vi "SRV_Motors Config Buttons MAP.vi"() -> (0 "error out":errorcluster)   [LabVIEW 2014]
doc: "A Producer-Consumer two-loop state machine template. This template uses the LPD Command Queues to drive its execution.\n\nThere are several advantages such as:\n- convenient error state control\n- the ability to pass data between states/loops/VIs via a variant\n- command history which is extremely valuable in troubleshooting when an error occurs\n\n\nAuthor: Mike Schultz\n\nLogicPD, Inc\nwww.logicpd.com"
uses:
  Support/SRV_Command-Data Queue Data Type.ctl
panel:
  in  "CLOSE":bool
  # "436x250"
  # "672x216"
  # "666x214"
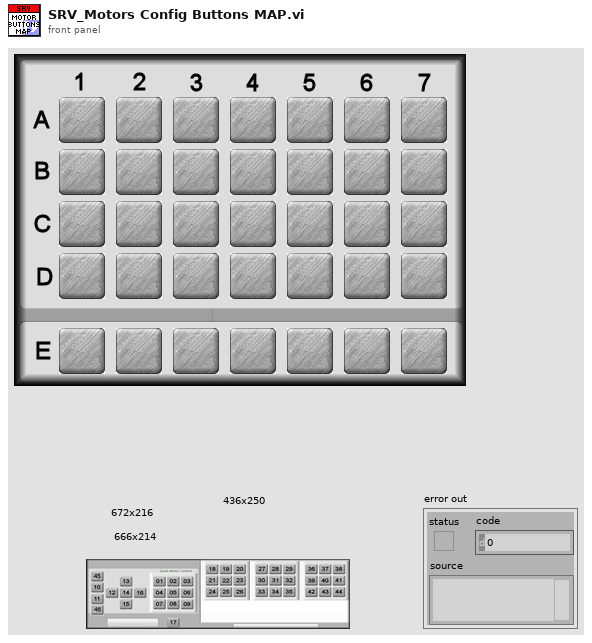
[diagram p1: front panel]
types:
  T1 = typedef "SRV_Command-Data Queue Data Type.ctl" = cluster{"Command":string, "Data":variant}
  T2 = cluster{"user event":refnum<user-event>, "VI ref":refnum<vi>}
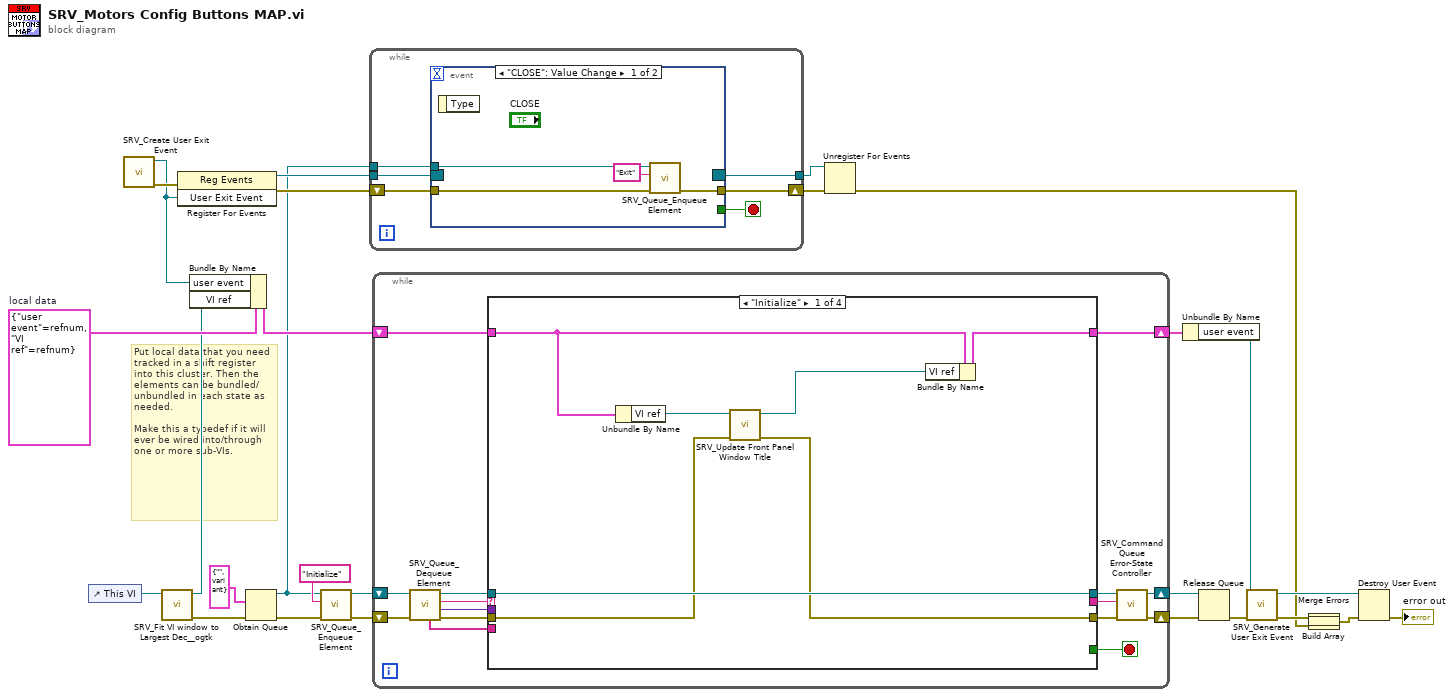
[diagram p0: block diagram]
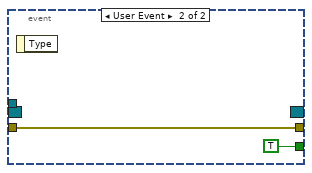
[diagram p2: hidden frame]
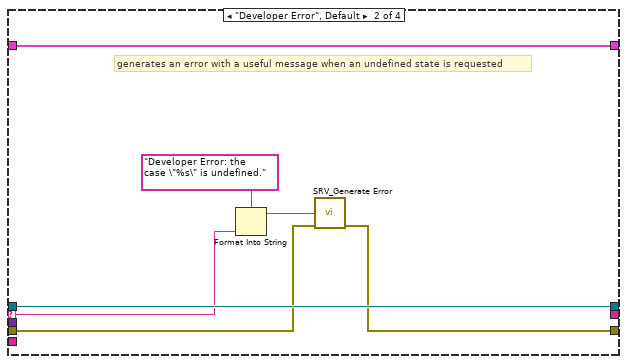
[diagram p3: hidden frame]
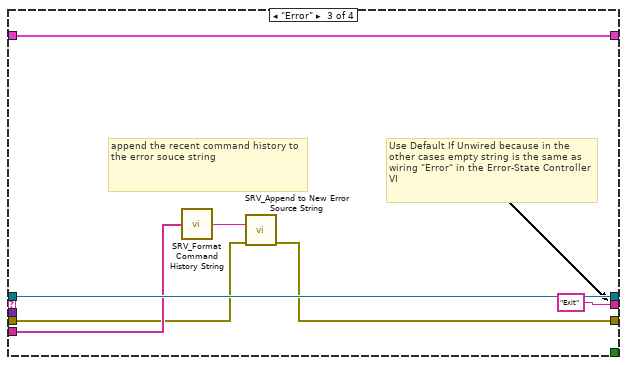
[diagram p4: hidden frame]
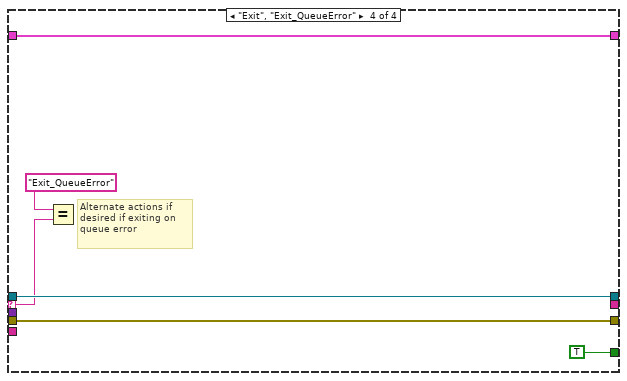
[diagram p5: hidden frame]
diagram:
  w21 = T2 {"user event"=refnum, "VI ref"=refnum}  # local data
  # "Put local data that you need tracked in a shift register into this cluster. Then the elements can be bundled/unbundled in each state as needed.\n\nMake this a typedef if it will ever be wired into/through one or more sub-VIs."
  n1 = control-ref of="This VI"() -> (w2:refnum<vi>)
  n2 = call "SRV_Create User Exit Event.vi"() -> ("error out"=w12:errorcluster, "User Exit Event"=w11:refnum<user-event>)  [unwired: 10 in]
  n3 = call "SRV_Fit VI window to Largest Dec__ogtk.vi"("VI Ref (calling VI)"=w2) -> ("error out"=w5:errorcluster, "dup VI Ref"=w1:refnum<vi>)  [unwired: 5 in]
  n4 = register-events(error in=w12, w11) -> (reference out=w28:refnum<event-registration>, error out=w27:errorcluster)  [unwired: 1 in]
  n5 = Bundle By Name(cluster=w21, "user event"=w11, "VI ref"=w1) -> (w20:T2)
  n6 = Obtain Queue(element data type=T1 {"Command"="", "Data"=variant} ("Queue Data Type"), error in (no error)=w5) -> (queue out=w7:refnum<queue>, error out=w8:errorcluster)  [unwired: 3 in, 1 out]
  n7 = call "SRV_Queue_Enqueue Element.vi"("error in (no error)"=w8, "Command"="Initialize", "Command-Data Queue"=w7) -> ("error out"=w3:errorcluster, "Command-Data Queue out"=w6:refnum<queue>)  [unwired: 6 in, 1 out]
  n8 = while {
    shift-right: [w33] -> w25
    shift-left: w27 -> [w34]
    tunnel: w7 -> [w32]
    tunnel: w28 -> [w31]
    tunnel: [w30] -> w26
    stop <- w29 stop-if-true
    n9 = event shown="[0] \"CLOSE\": Value Change" {
      selector: w31 -> [_ _]
      dyn-events: [_ _] -> w30
      timeout: _ -> [_ _]
      tunnel: w34 -> [w36 w40]
      tunnel: [w37 w40] -> w33
      tunnel: w32 -> [w35 _]
      tunnel: [_ TRUE] -> w29
      event "CLOSE": Value Change {
        n10 = event-data() -> ()  [unwired: 1 in, 1 out]
        n11 = call "SRV_Queue_Enqueue Element.vi"("error in (no error)"=w36, "Command"="Exit", "Command-Data Queue"=w35) -> ("error out"=w37:errorcluster)  [unwired: 6 in, 2 out]
      }
      event User Event {
        n12 = event-data() -> ()  [unwired: 1 in, 1 out]
      }
    }
  }
  n13 = while {
    shift-right: [w49] -> w24
    shift-left: w3 -> [w55]
    shift-right: [w47] -> w23
    shift-left: w6 -> [w53]
    shift-right: [w41] -> w19
    shift-left: w20 -> [w42]
    stop <- w43 stop-if-true
    n14 = call "SRV_Queue_Dequeue Element.vi"("error in (no error)"=w55, "Command-Data Queue"=w53) -> ("error out"=w54:errorcluster, "Data"=w46:variant, "Command"=w51:string, "Command-Data Queue out"=w52:refnum<queue>, "Command History"=w45:string[])  [unwired: 4 in, 1 out]
    n15 = case shown="\"Initialize\"" w51 {
      selector: w51 -> [_ w67 _ w79]
      tunnel: w54 -> [w61 w65 w71 w81]
      tunnel: [w60 w64 w72 w81] -> w50
      tunnel: w52 -> [w62 w69 w76 w82]
      tunnel: [w62 w69 w76 w82] -> w48
      tunnel: w46 -> [_ _ _ _]
      tunnel: w45 -> [_ _ w75 _]
      tunnel: [_ _ "Exit" ("Error Command") _] -> w44
      tunnel: [_ _ _ TRUE] -> w43
      tunnel: w42 -> [w58 w66 w73 w77]
      tunnel: [w57 w66 w73 w77] -> w41
      frame "Initialize" {
        n16 = Unbundle By Name(w58) -> ("VI ref"=w59:refnum<vi>)
        n17 = call "SRV_Update Front Panel Window Title.vi"("error in (no error)"=w61, "VI ref"=w59) -> ("error out"=w60:errorcluster, "VI ref out"=w56:refnum<vi>)  [unwired: 8 in]
        n18 = Bundle By Name(cluster=w58, "VI ref"=w56) -> (w57:T2)
      }
      frame "Developer Error", Default {
        # "generates an error with a useful message when an undefined state is requested"
        n19 = Format Into String(format string="Developer Error: the case \"%s\" is undefined.", w67) -> (resulting string=w63:string)  [unwired: 2 in, 1 out]
        n20 = call "SRV_Generate Error.vi"("Message"=w63, "error in (no error)"=w65) -> ("error out"=w64:errorcluster)  [unwired: 13 in]
      }
      frame "Error" {
        # "Use Default If Unwired because in the other cases empty string is the same as wiring \"Error\" in the Error-State Controller VI"
        # "append the recent command history to the error souce string"
        n21 = call "SRV_Format Command History String.vi"("Command History"=w75) -> ("Command History String"=w70:string)  [unwired: 14 in]
        n22 = call "SRV_Append to New Error Source String.vi"("Message String to append"=w70, "Error In (no error)"=w71) -> ("error out"=w72:errorcluster)  [unwired: 13 in]
      }
      frame "Exit", "Exit_QueueError" {
        # "Alternate actions if desired if exiting on queue error"
        n23 = Equal?(x="Exit_QueueError", y=w79) -> ()  [unwired: 1 out]
      }
    }
    n24 = call "SRV_Command Queue Error-State Controller.vi"("error in (no error)"=w50, "Error Command"=w44, "Command-Data Queue"=w48) -> ("error out"=w49:errorcluster, "Command-Data Queue out"=w47:refnum<queue>)  [unwired: 7 in]
  }
  n25 = Unregister For Events(event registration refnum=w26, error in=w25) -> (error out=w14:errorcluster)
  n26 = Unbundle By Name(w19) -> ("user event"=w18:refnum<user-event>)
  n27 = Release Queue(queue=w23, error in (no error)=w24) -> (error out=w17:errorcluster)  [unwired: 1 in, 2 out]
  n28 = call "SRV_Generate User Exit Event.vi"("error in (no error)"=w17, "User Exit Event"=w18) -> ("error out"=w15:errorcluster, "User Exit Event out"=w16:refnum<user-event>)  [unwired: 8 in]
  n29 = Build Array(w15, w14) -> (w10:errorcluster[])
  n30 = Merge Errors(w10) -> (w13:errorcluster)
  n31 = Destroy User Event(user event=w16, error in=w13) -> (error out=→"error out":errorcluster)
